vi "generatePermTrials.vi"(11 "semicolon seperated stimuli":string) -> (2 "max value":i32, 3 "perfmutated trials":string[](array[string]))   [LabVIEW 2014]
uses:
  <vilib>/Analysis/1siggen.llb/Riffle Array (I32).vi
  <vilib>/Analysis/NI_AALBase.lvlib
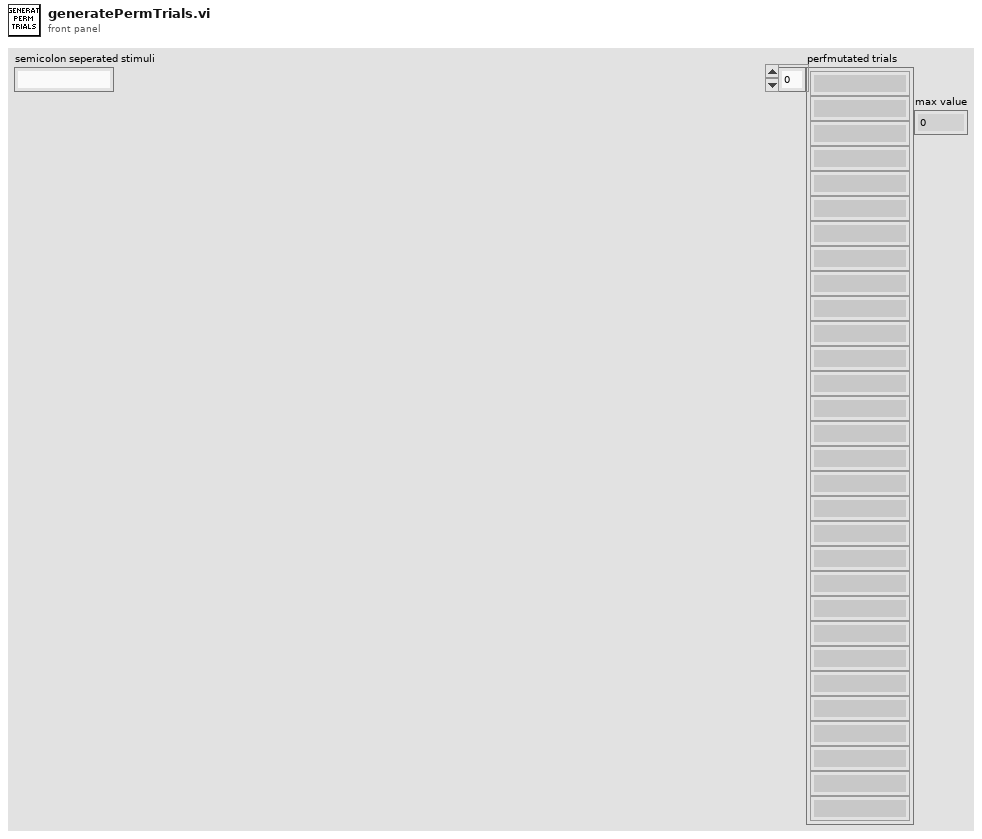
[diagram p1: front panel]
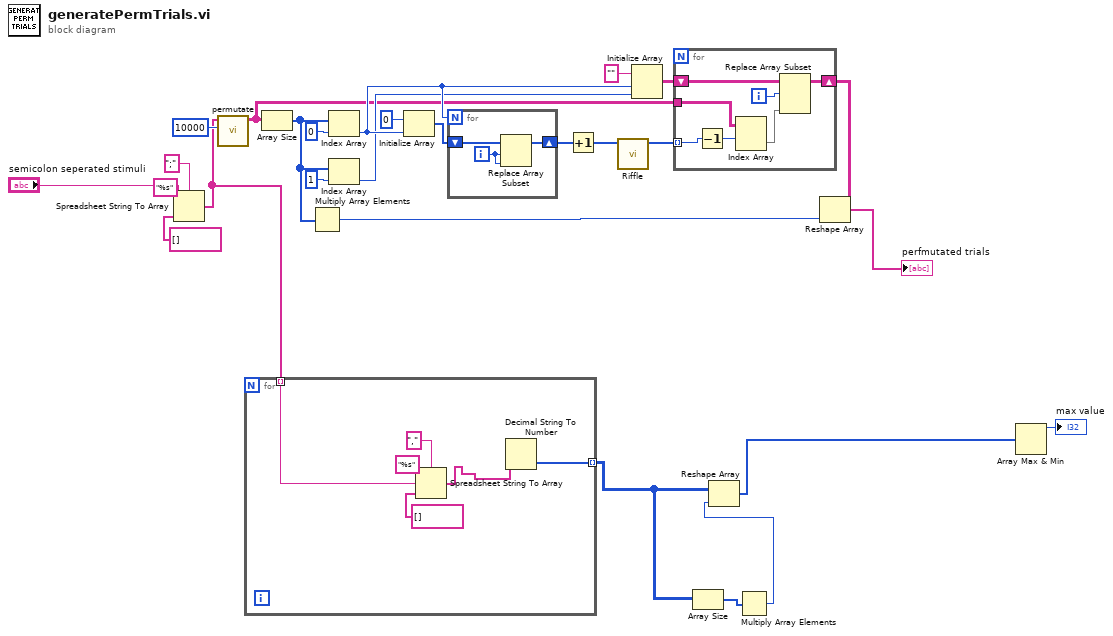
[diagram p0: block diagram]
diagram:
  n1 = Spreadsheet String To Array(delimiter (Tab)=";", format string="%s", spreadsheet string="semicolon seperated stimuli", array type (2D Dbl)=string[] []) -> (array=w6:string[])
  n2 = call "permutate.vi"("PermutationsLimit"=10000, "Input"=w6) -> ("Permutations"=w13:string[][])  [unwired: 9 in]
  n3 = for {
    tunnel: w6 -> [w30] mode=indexing
    tunnel: [w28] -> w3 mode=indexing
    n4 = Spreadsheet String To Array(delimiter (Tab)=",", format string="%s", spreadsheet string=w30, array type (2D Dbl)=string[] []) -> (array=w29:string[])
    n5 = Decimal String To Number(string=w29) -> (number=w28:i32[])  [unwired: 2 in, 1 out]
  }
  n6 = Array Size(array=w13) -> (size(s)=w12:i32[])
  n7 = Multiply Array Elements(1:w12) -> (0:w11:i32)
  n8 = Index Array(array=w12, index=0) -> (element=w18:i32)
  n9 = Index Array(array=w12, index=1) -> (element=w16:i32)
  n10 = Initialize Array(0, w18) -> (w22:i32[])
  n11 = for {
    N: w18 -> [_]
    shift-right: [w34] -> w21
    shift-left: w22 -> [w36]
    i -> [w35]
    n12 = Replace Array Subset(array=w36, new element=w35, index=w35) -> (w34:i32[])
  }
  n13 = Increment(x=w21) -> (x+1=w20:i32[])
  n14 = call-poly <vilib>:"Riffle.vi"("X"=w20) -> ("Riffled {X}"=w19:i32[])  [unwired: 8 in, 2 out]
  n15 = Initialize Array("", w18, w16) -> (w15:string[][])
  n16 = for {
    tunnel: w19 -> [w40] mode=indexing
    tunnel: w13 -> [w43]
    shift-right: [w38] -> w10
    shift-left: w15 -> [w41]
    i -> [w42]
    n17 = Decrement(x=w40) -> (x-1=w39:i32)
    n18 = Index Array(array=w43, index (row)=w39) -> (element=w37:string[])  [unwired: 1 in]
    n19 = Replace Array Subset(array=w41, new element=w37, index (row)=w42) -> (w38:string[][])  [unwired: 1 in]
  }
  n20 = Array Size(array=w3) -> (size(s)=w2:i32[])
  n21 = Multiply Array Elements(1:w2) -> (0:w1:i32)
  n22 = Reshape Array(w3, w1) -> (w5:i32[])
  n23 = Reshape Array(w10, w11) -> (→"perfmutated trials":string[])
  n24 = Array Max & Min(array=w5) -> (max value=→"max value":i32)  [unwired: 3 out]
